vi "testStringIncluded.vi"() -> ()   [LabVIEW 2019, in "AssertionTest.lvlib" / "AssertStringNotContainsString.lvlib"]
uses:
  AssertStringNotContainsString.lvlib
  Assertion/Assertion.lvlib
panel:
  out "error out":errorcluster
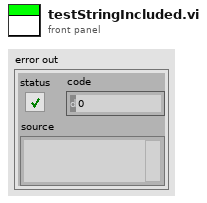
[diagram p1: front panel]
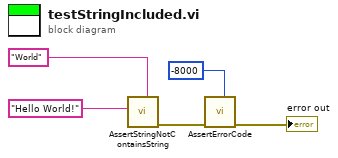
[diagram p0: block diagram]
diagram:
  n1 = call "AssertStringNotContainsString.vi"("Needle"="World", "Haystack"="Hello World!") -> ("error out"=w3:errorcluster)  [unwired: 9 in]
  n2 = call "AssertErrorCode.vi"("Expected"=-8000, "error in (no error)"=w3) -> ("error out"=→"error out":errorcluster)  [unwired: 9 in]
